vi "FIle_Show.vi"(8 "error in":errorcluster, 11 "File.lvclass (IN)":refnum<class "File.lvclass">) -> (0 "error out":errorcluster, 2 "File":T1, 3 "File.lvclass (OUT)":refnum<class "File.lvclass">)   [LabVIEW 2013, in "File.lvclass"]
uses:
  File.lvclass
  File.lvclass/File.ctl
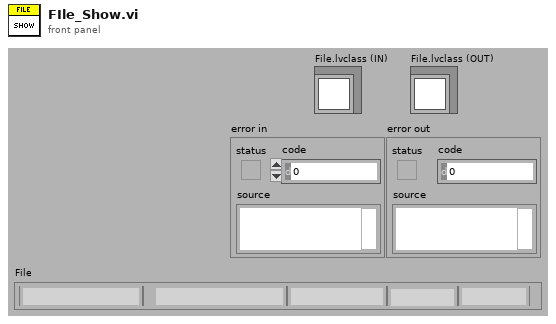
[diagram p1: front panel]
types:
  T1 = cluster{"Name":string, "Path":path, "Version":string, "Start Tiime":string, "Stop Tiime":string}
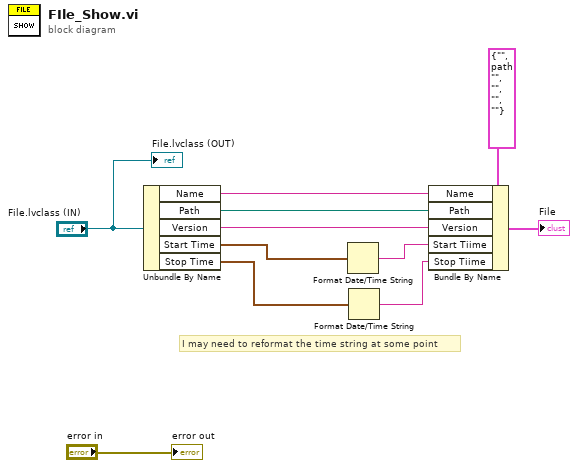
[diagram p0: block diagram]
diagram:
  # "I may need to reformat the time string at some point"
  n1 = Unbundle By Name("File.lvclass (IN)") -> ("Name"=w9:string, "Path"=w6:path, "Version"=w7:string, "Start Time"=w4:timestamp, "Stop Time"=w3:timestamp)
  n2 = Format Date/Time String(seconds (now)=w4) -> (date/time string=w2:string)  [unwired: 2 in]
  n3 = Format Date/Time String(seconds (now)=w3) -> (date/time string=w1:string)  [unwired: 2 in]
  n4 = Bundle By Name(cluster=T1 {"Name"="", "Path"=path "", "Version"="", "Start Tiime"="", "Stop Tiime"=""} ("File"), "Name"=w9, "Path"=w6, "Version"=w7, "Start Tiime"=w2, "Stop Tiime"=w1) -> (→"File":T1)
  "File.lvclass (OUT)" <- "File.lvclass (IN)"
  "error out" <- "error in"
